vi "Upload IOT Datavi.vi"   [LabVIEW 2017]
uses:
  SfisTestOcx/sifi process.ctl
  Sqlite/CBB/CreatTable.vi
  Sqlite/CBB/ReadAllData.vi
  Sqlite/CBB/InsertRowData.vi
  Sqlite/SQLite.lvlib
types:
  T1 = typedef "提取参数项目.ctl" = enum16{"初始化", "基准拍照点提取", "物理距离信息提取", "锁附总表参数提取", "图纸锁附坐标提取", "更新图面offset", "图纸投影至机械", "提取数据"}
  T2 = typedef "sifi process.ctl" = enum16{"standby", "sifi initial", "check route", "get version", "upload result", "initial register"}
  T3 = typedef "IOT数据更新选项.ctl" = enum16{"初始化", "更新数据", "获取寄存器", "前后站信息交互", "更新前站inflow&barcode"}
  T4 = cluster{"IOT":cluster{"table":string, "column":string[]}, "ER":cluster{"table":string, "column":string[]}}
  T5 = typedef "计算时间控件.ctl" = cluster{"前侧ct":cluster{"start time":i32, "end time":i32, "ct":i32}, "后侧ct":cluster{"start time":i32, "end time":i32, "ct":i32}, "wait time":cluster{"start time":i32, "end time":i32, "ct":i32}}
  T6 = typedef "sifi state output.ctl" = cluster{"initial ok":bool, "login ok":bool, "logout ok":bool, "check route":bool, "update ok":bool, "get versionOK":bool}
  T7 = cluster{"%Y_%m_%d_%H_%M_%S%3u":string, "%Y_%m_%d":string, "%H_%M_%S%3u":string}
  T8 = typedef "参数集合.ctl" = cluster{"主&辅助定位孔拍照位置":T9, "物距提取信息":T11, "锁附总表参数":T14, "图面投影后检索结果":T19}
  T9 = typedef "主&辅助定位孔拍照位置.ctl" = cluster{"主定位孔拍照位置":T10, "辅助定位孔拍照位置":T10}
  T10 = typedef "定位孔拍照位置.ctl" = cluster{"动子位置":dbl, "供料轴位置":dbl, "Z轴位置":dbl}
  T11 = typedef "物距提取信息.ctl" = cluster{"物距":T12, "橡皮泥标记点":T10, "物距文档检索状态":T13, "标记拍照Z轴":dbl}
  T12 = typedef "物理距离.ctl" = cluster{"动子方向":dbl, "供料轴方向":dbl}
  T13 = typedef "总表检索状态.ctl" = enum16{"检索点位顺序超出范围", "检索OK"}
  T14 = typedef "锁附参数.ctl" = cluster{"锁附扭力":dbl, "锁附位置参数":T15, "锁附速度":T16, "锁附检测类参数":T17, "锁附点位编号":string, "总表检索状态":T13, "锁附总颗数":dbl, "起子编号":T18, "顺序编号":dbl, "组装孔？":bool, "扭力offset":dbl, "设定扭力":dbl, "锁附自救屏蔽？":bool}
  T15 = typedef "锁附位置参数.ctl" = cluster{"动子位置":dbl, "供料轴位置":dbl, "阶梯高度位置":dbl, "锁附深度":dbl}
  T16 = typedef "锁附速度.ctl" = cluster{"驱动速度":dbl, "加速度":dbl}
  T17 = typedef "锁附检测类参数.ctl" = cluster{"报警功能屏蔽？":bool, "锁附设定时间":dbl, "浮锁检测高度":dbl, "浮锁检测容差":dbl}
  T18 = typedef "起子编号.ctl" = enum16{"NA", "driver01", "driver02", "driver03", "driver04"}
  T19 = typedef "图面投影后检索结果.ctl" = cluster{"图纸投影后点位坐标":T12, "图面投影后文件检索状态":T13, "offset获取辅助集合":T20}
  T20 = typedef "offset获取辅助集合.ctl" = cluster{"offset获取半径spec":T21, "拍照高度":dbl, "曝光时间":dbl}
  T21 = typedef "上下限.ctl" = cluster{"上限":dbl, "下限":dbl}
  T22 = typedef "螺丝机IOT数据信息.ctl" = cluster{"IOT基本信息":T23, "扭力":string[]}
  T23 = typedef "IOT数据基本信息.ctl" = cluster{"number":string, "ID":string, "Version":string, "Date":string, "Time":string, "Device SN":string, "Carrier SN":string, "Inflow":string, "Work":string, "Wait":string, "Outflow":string, "SFIS":string, "Alignment Times":string, "Press1":string, "ifsyn":string}
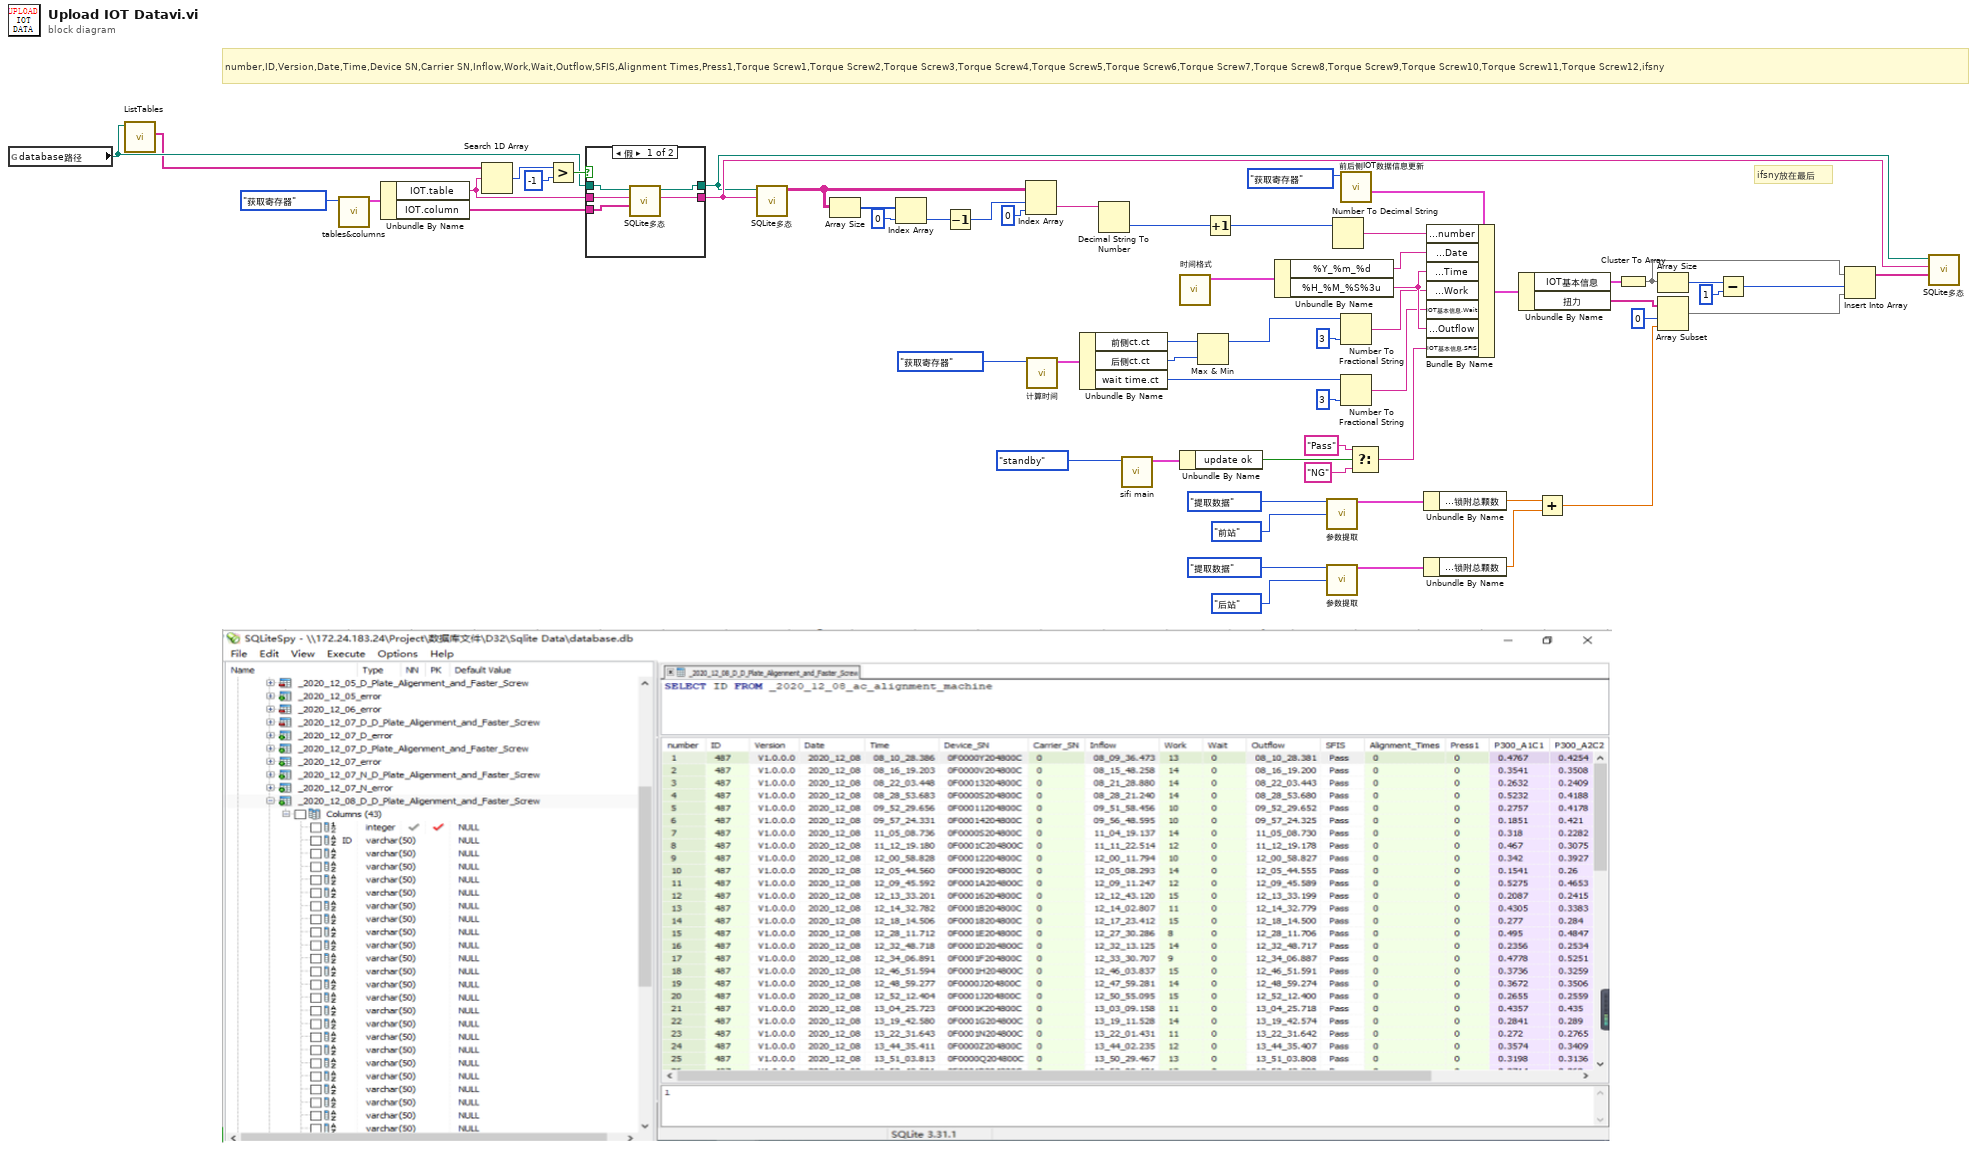
[diagram p0: block diagram]
diagram:
  # "number,ID,Version,Date,Time,Device SN,Carrier SN,Inflow,Work,Wait,Outflow,SFIS,Alignment Times,Press1,Torque Screw1,Torque Screw2,Torque Screw3,Torque Screw4,Torque Screw5,Torque Screw6,Torque Screw7,Torque Screw8,Torque Screw9,Torque Screw10,Torque Screw11,Torque Screw12,ifsny"
  # "ifsny放在最后"
  n1 = global read "数据库全局.vi" "database路径"() -> (w32:path)
  n2 = call "ListTables.vi"("DbPath"=w32) -> ("Tables"=w1:string[])  [unwired: 7 in, 3 out]
  n3 = call "tables&columns.vi"("选项"=enum16{"初始化", "获取寄存器"}."获取寄存器") -> ("Tables&columns"=w31:T4)  [unwired: 9 in, 1 out]
  n4 = Unbundle By Name(w31) -> ("IOT.table"=w49:string, "IOT.column"=w33:string[])
  n5 = Search 1D Array(1D array=w1, element=w49) -> (index of element=w46:i32)  [unwired: 1 in]
  n6 = Greater?(x=w46, y=-1) -> (0:w48:bool)
  n7 = case shown="假" w48 {
    tunnel: w32 -> [w66 w68]
    tunnel: w49 -> [w65 w67]
    tunnel: w33 -> [w64 _]
    tunnel: [w63 w68] -> w50
    tunnel: [w62 w67] -> w51
    frame False {
      n8 = call-poly "SQLite多态.vi"("Columns"=w64, "Table Name"=w65, "DbPath"=w66) -> ("Table Name out"=w62:string, "DbPath out"=w63:path)  [unwired: 6 in, 1 out]
    }
    frame True {
    }
  }
  n9 = call-poly "SQLite多态.vi"("Table Name"=w51, "DbPath"=w50) -> ("Results"=w58:string[][])  [unwired: 4 in, 5 out]
  n10 = Array Size(array=w58) -> (size(s)=w53:i32[])
  n11 = Index Array(array=w53, index=0 ("索引")) -> (element=w55:i32)
  n12 = Decrement(x=w55) -> (x-1=w56:i32)
  n13 = Index Array(array=w58, index (row)=w56, index (col)=0 ("禁用的索引 (列)")) -> (element=w59:string)
  n14 = call "计算时间.vi"("选项"=enum16{"初始化", "更新数据", "获取寄存器"}."获取寄存器") -> ("计算时间"=w27:T5)  [unwired: 10 in]
  n15 = Unbundle By Name(w27) -> ("前侧ct.ct"=w22:i32, "后侧ct.ct"=w21:i32, "wait time.ct"=w23:i32)
  n16 = Decimal String To Number(string=w59) -> (number=w57:i32)  [unwired: 2 in, 1 out]
  n17 = call "sifi main.vi"("sifi process"=sifi_process."standby") -> ("sifi state output"=w41:T6)  [unwired: 8 in, 2 out]
  n18 = call "时间格式.vi"() -> ("时间格式"=w37:T7)  [unwired: 11 in]
  n19 = Unbundle By Name(w41) -> ("update ok"=w42:bool)
  n20 = Max & Min(x=w22, y=w21) -> (max(x,y)=w20:i32)  [unwired: 1 out]
  n21 = Increment(x=w57) -> (x+1=w60:i32)
  n22 = Unbundle By Name(w37) -> ("%Y_%m_%d"=w38:string, "%H_%M_%S%3u"=w39:string)
  n23 = call "参数提取.vi"("提取参数项目"=提取参数项目."提取数据", "前/后站"=enum16{"前站", "后站"}."前站") -> ("参数集合out"=w11:T8)  [unwired: 10 in, 3 out]
  n24 = call "参数提取.vi"("提取参数项目"=提取参数项目."提取数据", "前/后站"=enum16{"前站", "后站"}."后站") -> ("参数集合out"=w5:T8)  [unwired: 10 in, 3 out]
  n25 = Number To Decimal String(number=w60) -> (decimal integer string=w61:string)  [unwired: 1 in]
  n26 = call "前后侧IOT数据信息更新.vi"("选项"=IOT数据更新选项."获取寄存器") -> ("后侧IOT数据信息"=w34:T22)  [unwired: 9 in, 1 out]
  n27 = Number To Fractional String(number=w20, precision (6)=i16 3 ("精度(6)")) -> (F-format string=w19:string)  [unwired: 2 in]
  n28 = Number To Fractional String(number=w23, precision (6)=i16 3 ("精度(6)")) -> (F-format string=w24:string)  [unwired: 2 in]
  n29 = Select(t="Pass" ("%H_%M_%S%3u"), s=w42, f="NG" ("%H_%M_%S%3u")) -> (s? t:f=w45:string)
  n30 = Unbundle By Name(w11) -> ("锁附总表参数.锁附总颗数"=w10:dbl)
  n31 = Unbundle By Name(w5) -> ("锁附总表参数.锁附总颗数"=w4:dbl)
  n32 = Bundle By Name(cluster=w34, "IOT基本信息.number"=w61, "IOT基本信息.Date"=w38, "IOT基本信息.Time"=w39, "IOT基本信息.Work"=w19, "IOT基本信息.Wait"=w24, "IOT基本信息.Outflow"=w39, "IOT基本信息.SFIS"=w45) -> (w14:T22)
  n33 = Unbundle By Name(w14) -> ("IOT基本信息"=w35:T23, "扭力"=w9:string[])
  n34 = Add(x=w10, y=w4) -> (x+y=w6:dbl)
  n35 = Cluster To Array(cluster=w35) -> (array=w18:string[])
  n36 = Array Size(array=w18) -> (size(s)=w17:i32)
  n37 = Array Subset(array=w9, index=0 ("索引"), length=w6) -> (w2:string[])
  n38 = Subtract(x=w17, y=1 ("x")) -> (x-y=w15:i32)
  n39 = Insert Into Array(array=w18, index=w15, new element=w2) -> (w36:string[])
  n40 = call-poly "SQLite多态.vi"("InsertData"=w36, "Table Name"=w51, "DbPath"=w50) -> ()  [unwired: 6 in, 3 out]
